vi "Get ClientID List.vi"(8 "error in (no error)":errorcluster, 11 "Server in":refnum<class "Server.lvclass">) -> (0 "error out":errorcluster, 2 "ClientIDs":string[](array[string]), 3 "Server out":refnum<class "Server.lvclass">)   [LabVIEW 2013, in "MQTT Server.lvlib" / "Server.lvclass"]
uses:
  Server.lvclass
  Server.lvclass/Server.ctl
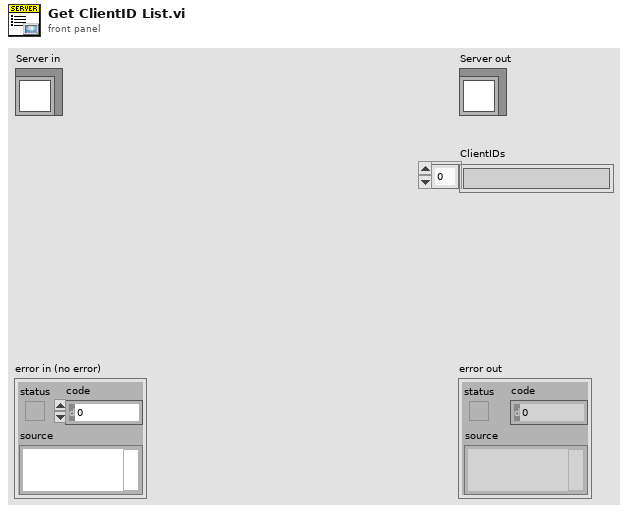
[diagram p1: front panel]
types:
  T1 = typedef "MQTT Server.lvlib/Server.lvclass/SessionRef -- cluster.ctl" = cluster{"ClientID":string, "SessionMailbox":refnum<queue>}
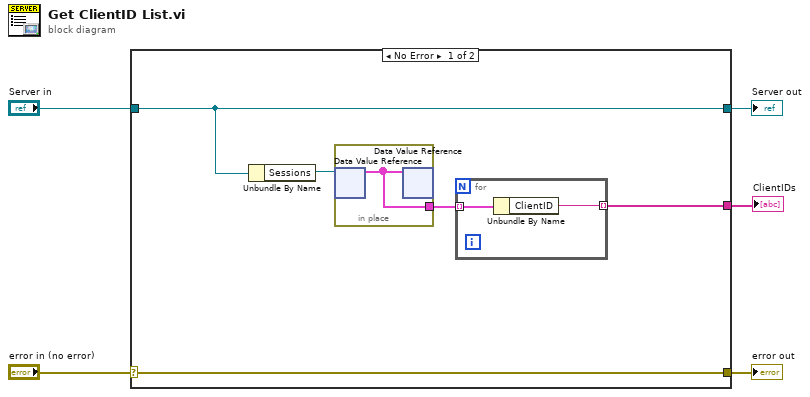
[diagram p0: block diagram]
diagram:
  n1 = case shown="No Error" "error in (no error)" {
    selector: "error in (no error)" -> [w10 w15]
    tunnel: [w10 w15] -> w4
    tunnel: [w9 w14] -> w2
    tunnel: "Server in" -> [w9 w14]
    tunnel: [w6 _] -> w1
    frame No Error {
      n2 = Unbundle By Name(w9) -> ("Sessions"=w8:refnum<data-value>)
      n3 = in-place {
        in-place-border: [w13] -> w7
        n4 = in-place-dvr #1(w8) -> (w13:T1[])  [unwired: 1 out]
        n5 = in-place-dvr #1(w13) -> ()  [unwired: 2 out]
      }
      n6 = for {
        tunnel: w7 -> [w12] mode=indexing
        tunnel: [w11] -> w6 mode=indexing
        n7 = Unbundle By Name(w12) -> ("ClientID"=w11:string)
      }
    }
    frame Error {
    }
  }
  "error out" <- w4
  "Server out" <- w2
  "ClientIDs" <- w1
